vi "Adapt To Type.vi"(6 "Nulls as Defaults (F)":bool, 7 "Type and Defaults":variant, 8 "error in (no error)":errorcluster, 11 "Variant in":variant) -> (0 "error out":errorcluster, 3 "Variant out":variant)   [LabVIEW 2020, in "JKI JSON Object Serialization.lvlib"]
doc: "Converts 'Variant in' to the type wired to 'Type and Defaults'. This VI copies values from elements within a cluster or object's private data to elements with the same name in another cluster or object. This works without accessor methods. \n\nGCraftsman JSON Object Serialization Toolkit\nwww.GCraftsman.com\nCopyright (c) 2017, GCraftsman"
uses:
  JKI JSON Object Serialization.lvlib
  Deserializer/Deserializer.lvclass
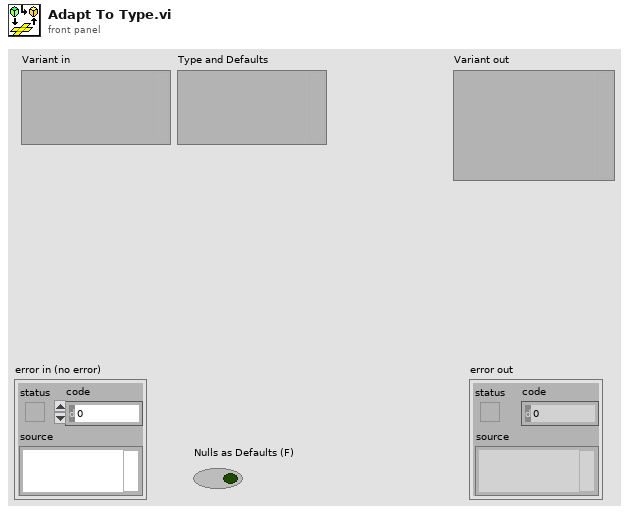
[diagram p1: front panel]
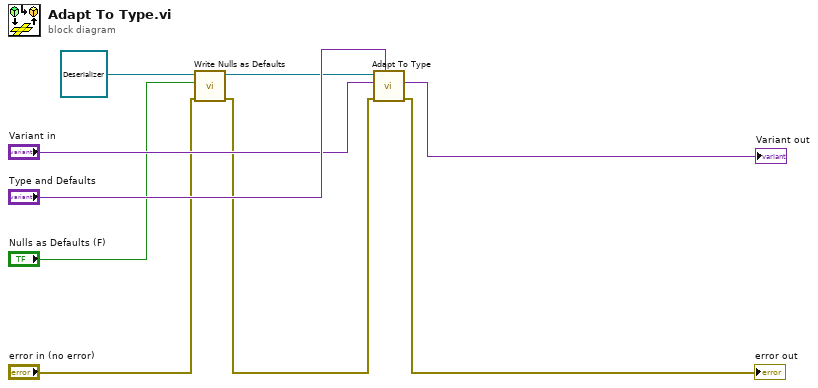
[diagram p0: block diagram]
diagram:
  n1 = call-dynamic "Write Nulls as Defaults.vi"("error in (no error)"="error in (no error)", "Nulls as Defaults"="Nulls as Defaults (F)", "JSON Deserializer in"=refnum<class "Deserializer.lvclass"> refnum ("JSON Object Deserializer.lvclass")) -> ("error out"=w3:errorcluster, "JSON Deserializer out"=w5:refnum<class "Deserializer.lvclass">)  [unwired: 7 in]
  n2 = call-dynamic "Adapt To Type.vi"("Type and Defaults"="Type and Defaults", "error in (no error)"=w3, "Variant in"="Variant in", "Deserializer in"=w5) -> ("error out"=→"error out":errorcluster, "Variant out"=→"Variant out":variant)  [unwired: 5 in, 1 out]
